vi "Create ObjectMap.vi"(5 "ObjectMap In":refnum<class "ObjectMap.lvclass">, 7 "Map Implementation (Variant Attributes)":refnum<class "MapImp.lvclass">, 8 "error in (no error)":errorcluster) -> (0 "error out":errorcluster, 3 "ObjectMap":refnum<class "ObjectMap.lvclass">)   [LabVIEW 2013, in "LapDog.Collections.v_.Maps.lvlib" / "ObjectMap.lvclass"]
doc: "Creates a new map object.\n\nTo use something other than the default implementation, connect the implementation's class constant to the Map Implementation terminal."
uses:
  ObjectMap.lvclass
  MapImp/MapImp.lvclass
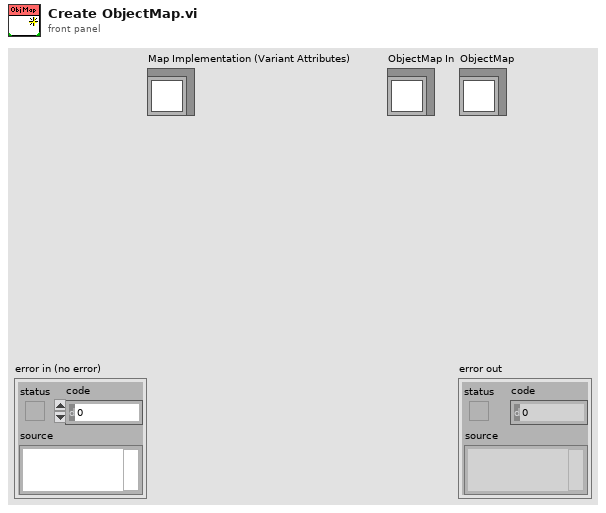
[diagram p1: front panel]
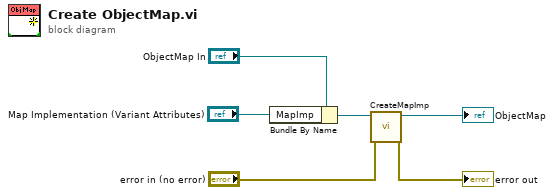
[diagram p0: block diagram]
diagram:
  n1 = Bundle By Name(cluster="ObjectMap In", "MapImp"="Map Implementation (Variant Attributes)") -> (w4:refnum<class "ObjectMap.lvclass">)
  n2 = call "CreateMapImp.vi"("error in (no error)"="error in (no error)", "Map in"=w4) -> ("error out"=→"error out":errorcluster, "Map out"=→"ObjectMap":refnum<class "ObjectMap.lvclass">)  [unwired: 8 in]
